vi "Shooter.vi"   [LabVIEW 2019]
uses:
  <vilib>/Rock Robotics/SystemInterfaces/DIO/FPGA_DIOPWMChannel.ctl
  <vilib>/Rock Robotics/WPI/Joystick/WPI_JoystickDeviceEnum.ctl
  <vilib>/Rock Robotics/WPI/Utilities/WPI_GetSetVariantRefNum.vi
  <vilib>/Rock Robotics/WPI/RobotDrive/WPI_RobotDriveOpen2MotorWithTalonSRX.vi
  <vilib>/Rock Robotics/WPI/MotorControl/WPI_MotorControlOpen TalonSRX.vi
types:
  T1 = typedef "WPI_JoystickDeviceEnum.ctl" = enum16{"USB 0", "USB 1", "USB 2", "USB 3", "USB 4", "USB 5"}
  T2 = typedef "FPGA_DIOPWMChannel.ctl" = enum8{"PWM 0", "PWM 1", "PWM 2", "PWM 3", "PWM 4", "PWM 5", "PWM 6", "PWM 7", "PWM 8", "PWM 9", "PWM MXP 0", "PWM MXP 1", "PWM MXP 2", "PWM MXP 3", "PWM MXP 4", "PWM MXP 5", "PWM MXP 6", "PWM MXP 7", "PWM MXP 8", "PWM MXP 9", "Invalid"}
  T3 = typedef "WPI_RobotDriveDevRef.ctl" = cluster{"DevStatus":errorcluster, "Motors[]":T4[], "Square Inputs":bool, "Max Output":dbl}
  T4 = typedef "WPI_MotorControlDeviceRef.ctl" = cluster{"DeviceStatus":errorcluster, "Type":T5, "PWM":cluster{"PWM Channel":T2, "DeadBand":T6}, "CAN":cluster{"Device Number":u8, "SetOutput VI Ref":variant, "GetOutput VI Ref":variant, "Enable VI Ref":variant, "Disable VI Ref":variant, "Data":variant}, "Invert":bool, "DIO PWM":cluster{"PWM \"Enable\" Channel":T2, "DIOChannel":T7, "PWM Rate":dbl}}
  T5 = typedef "WPI_MotorControlType.ctl" = enum16{"PWM", "CAN", "DIO PWM"}
  T6 = typedef "WPI_PWMDeadband.ctl" = cluster{"Name":string, "maxPositivePwm":i32, "minPositivePwm":i32, "centerPwm":i32, "maxNegativePwm":i32, "minNegativePwm":i32, "angularRange":u16}
  T7 = typedef "FPGA_DIOChannel.ctl" = enum8{"DIO 0", "DIO 1", "DIO 2", "DIO 3", "DIO 4", "DIO 5", "DIO 6", "DIO 7", "DIO 8", "DIO 9", "DIO MXP 0", "DIO MXP 1", "DIO MXP 2", "DIO MXP 3", "DIO MXP 4", "DIO MXP 5", "DIO MXP 6", "DIO MXP 7", "DIO MXP 8", "DIO MXP 9", "DIO MXP 10", "DIO MXP 11", "DIO MXP 12", "DIO MXP 13", "DIO MXP 14", "DIO MXP 15", "SPI Port CS1", "SPI Port CS2", "SPI Port CS3", "SPI Port MISO", "SPI Port MOSI", "Invalid"}
  T8 = typedef "WPI_JoystickDevRef.ctl" = cluster{"Device":T1}
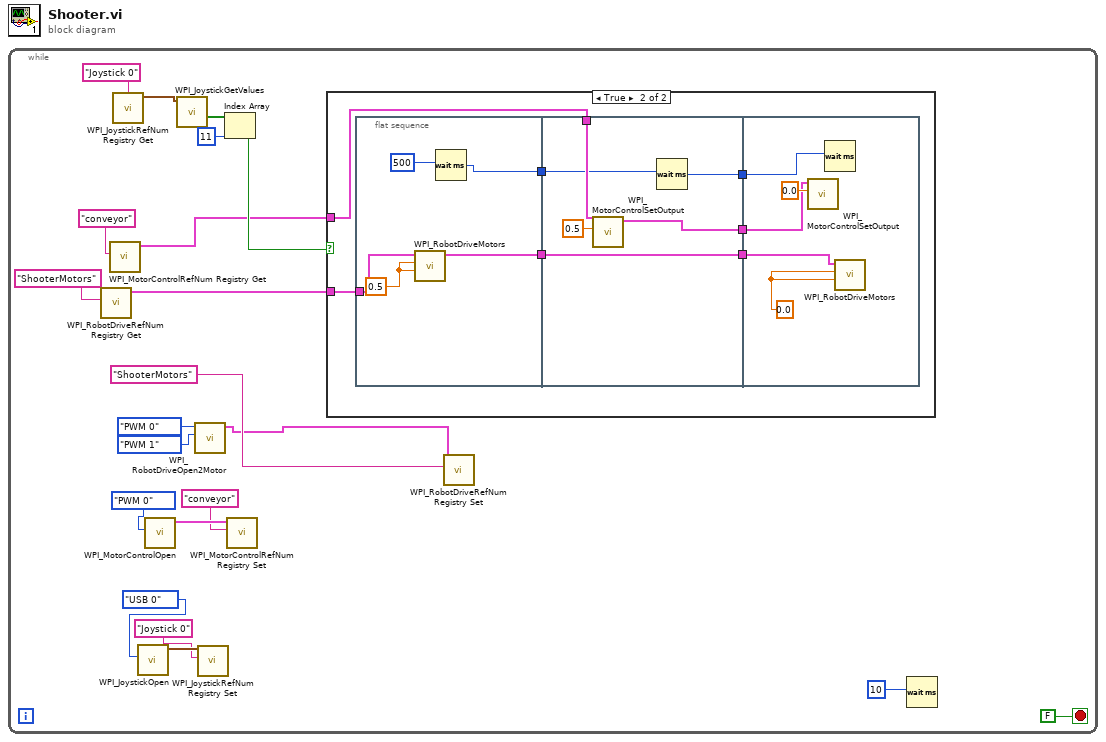
[diagram p0: block diagram]
diagram:
  n1 = while {
    stop <- FALSE stop-if-true
    n2 = call <vilib>:"WPI_RobotDriveRefNum Registry Get.vi"("refnum name"="ShooterMotors") -> ("RobotDriveDevRef"=w12:T3)  [unwired: 9 in, 1 out]
    n3 = call <vilib>:"WPI_MotorControlRefNum Registry Get.vi"("refnum name"="conveyor") -> ("MotorControlDevRef"=w13:T4)  [unwired: 9 in, 1 out]
    n4 = call <vilib>:"WPI_JoystickRefNum Registry Get.vi"("refnum name"="Joystick 0") -> ("JoystickDevRef"=w20:T8)  [unwired: 9 in, 1 out]
    n5 = call <vilib>:"WPI_JoystickOpen.vi"("JoystickDevice"=WPI_JoystickDeviceEnum."USB 0") -> ("JoystickDevRef"=w9:T8)  [unwired: 10 in]
    n6 = call-poly <vilib>:"WPI_MotorControlOpen.vi"("PWM Channel"=FPGA_DIOPWMChannel."PWM 0") -> ("MotorControlDeviceRef"=w10:T4)  [unwired: 9 in, 1 out]
    n7 = call <vilib>:"WPI_JoystickGetValues.vi"("JoystickDevRef"=w20) -> ("Buttons"=w18:bool[])  [unwired: 6 in, 4 out]
    n8 = call-poly <vilib>:"WPI_RobotDriveOpen2Motor.vi"("Right Motor"=FPGA_DIOPWMChannel."PWM 1", "Left Motor"=FPGA_DIOPWMChannel."PWM 0") -> ("RobotDriveDevRef"=w1:T3)  [unwired: 8 in, 1 out]
    n9 = call <vilib>:"WPI_JoystickRefNum Registry Set.vi"("refnum name"="Joystick 0", "JoystickDevRef"=w9) -> ()  [unwired: 8 in, 2 out]
    n10 = Index Array(array=w18, index=11) -> (element=w16:bool)
    n11 = call <vilib>:"WPI_MotorControlRefNum Registry Set.vi"("refnum name"="conveyor", "MotorControlDevRef"=w10) -> ()  [unwired: 8 in, 2 out]
    n12 = case shown="True" w16 {
      tunnel: w13 -> [_ w28]
      tunnel: w12 -> [_ w27]
      frame False {
      }
      frame True {
        n13 = flat-sequence {
          tunnel: w27 -> [w33]
          tunnel: [w30] -> w26
          tunnel: [w29] -> w22
          tunnel: w28 -> [w39]
          tunnel: w26 -> [w37]
          tunnel: [w37] -> w25
          tunnel: [w36] -> w24
          tunnel: [w35] -> w23
          tunnel: w22 -> [w34]
          tunnel: w25 -> [w43]
          tunnel: w24 -> [w41]
          tunnel: w23 -> [w40]
          frame #0 {
            w32 = 0.5 ("LeftSpeed")
            n14 = call <vilib>:"WPI_RobotDriveMotors.vi"("RightSpeed"=w32, "LeftSpeed"=w32, "RobotDriveDevRef"=w33) -> ("RobotDriveDevRef"=w30:T3)  [unwired: 6 in, 2 out]
            n15 = Wait (ms)(milliseconds to wait=u32 500 ("millisecond timer value")) -> (millisecond timer value=w29:u32)
          }
          frame #1 {
            n16 = call <vilib>:"WPI_MotorControlSetOutput.vi"("Output"=0.5, "MotorControlDevRef"=w39) -> ("MotorControlDevRef"=w36:T4)  [unwired: 7 in, 2 out]
            n17 = Wait (ms)(milliseconds to wait=w34) -> (millisecond timer value=w35:u32)
          }
          frame #2 {
            w44 = 0.0 ("LeftSpeed")
            n18 = call <vilib>:"WPI_MotorControlSetOutput.vi"("Output"=0.0, "MotorControlDevRef"=w41) -> ()  [unwired: 7 in, 3 out]
            n19 = Wait (ms)(milliseconds to wait=w40) -> ()  [unwired: 1 out]
            n20 = call <vilib>:"WPI_RobotDriveMotors.vi"("RightSpeed"=w44, "LeftSpeed"=w44, "RobotDriveDevRef"=w43) -> ()  [unwired: 6 in, 3 out]
          }
        }
      }
    }
    n21 = call <vilib>:"WPI_RobotDriveRefNum Registry Set.vi"("refnum name"="ShooterMotors", "RobotDriveDevRef"=w1) -> ()  [unwired: 8 in, 2 out]
    n22 = Wait (ms)(milliseconds to wait=u32 10 ("millisecond timer value")) -> ()  [unwired: 1 out]
  }
